vi "Wave1D_Solver.vi"(0 "F(t, x)":dbl[][](array[numeric]), 1 "Initial Value":dbl[](array[numeric]), 2 "Initial Derivative":dbl[](array[numeric]), 5 "k":dbl=1.0, 7 "a":dbl, 9 "Domain":T2={"t"={"initial t"=0.0, "final t"=1.0, "# of t-points"=11}, "x"={"start x"=0.0, "end x"=1.0, "# of x-points"=11}}, 11 "error in (no error)":errorcluster, 12 "Boundary Condition":cluster{"type":T1, "Value":dbl[]}[](array[cluster]) {"type" items=["Dirichlet", "Neumann"]}) -> (4 "U(t, x)":dbl[][](array[numeric]), 15 "error out":errorcluster)   [LabVIEW 2017, in "NI_PDE.lvlib"]
uses:
  <vilib>/gmath/NI_PDE.lvlib
  <vilib>/gmath/pde.llb/Common/PDE_BC Type.ctl
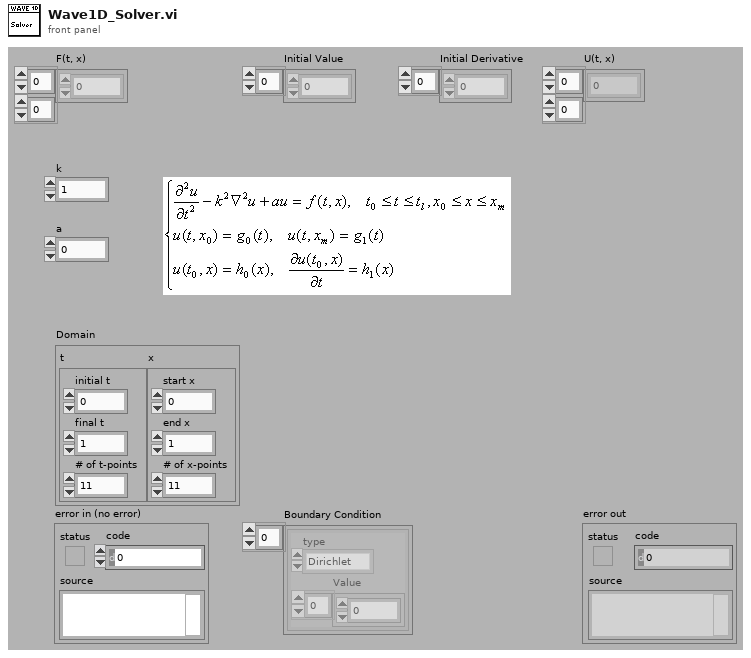
[diagram p1: front panel]
types:
  T1 = typedef "NI_PDE.lvlib/PDE_BC Type.ctl" = i32
  T2 = cluster{"t":cluster{"initial t":dbl, "final t":dbl, "# of t-points":i32}, "x":cluster{"start x":dbl, "end x":dbl, "# of x-points":i32}}
  T3 = typedef "NI_PDE.lvlib/Wave1D_Data.ctl" = cluster{"PDE":cluster{"k":dbl, "a":dbl, "F(t, x)":dbl[][]}, "Domain":cluster{"t":cluster{"initial t":dbl, "final t":dbl, "# of t-points":i32}, "x":cluster{"start x":dbl, "end x":dbl, "# of x-points":i32}, "delta":cluster{"delta t":dbl, "delta x":dbl}}, "BC":cluster{"Start X":cluster{"type":T1, "Value":dbl[]}, "End X":cluster{"type":T1, "Value":dbl[]}}, "IC":cluster{"Value":dbl[], "Derivative":dbl[]}, "A":cluster{"Sub Diag":dbl[], "Diag":dbl[], "Super Diag":dbl[], "A":T4}, "LU of A":cluster{"L":dbl[], "U":cluster{"Diag":dbl[], "Super Diag":dbl[], "2nd Super Diag":dbl[]}, "Pivot":i32[]}, "State":cluster{"U":dbl[], "AU":dbl[], "Old AU":dbl[], "start index":i32, "length":i32}}
  T4 = typedef "NI_Matrix.lvlib/RealMatrix.ctl" = dbl[][]
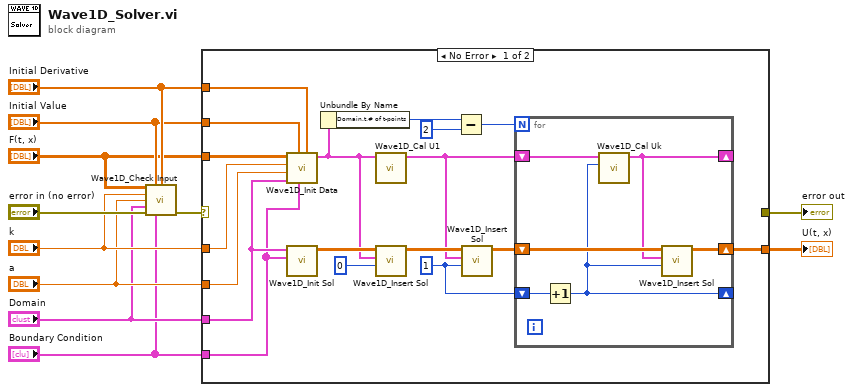
[diagram p0: block diagram]
diagram:
  n1 = call <vilib>:"Wave1D_Check Input.vi"("F(t, x)"="F(t, x)", "Initial Value"="Initial Value", "Initial Derivative"="Initial Derivative", "k"="k", "a"="a", "Domain"="Domain", "error in (no error)"="error in (no error)", "Boundary Condition"="Boundary Condition") -> ("error out"=w10:errorcluster)  [unwired: 7 out]
  n2 = case shown="No Error" w10 {
    selector: w10 -> [_ w36]
    tunnel: "Initial Derivative" -> [w28 _]
    tunnel: "Initial Value" -> [w29 _]
    tunnel: "F(t, x)" -> [w27 _]
    tunnel: "k" -> [w26 _]
    tunnel: "a" -> [w25 _]
    tunnel: "Domain" -> [w24 _]
    tunnel: "Boundary Condition" -> [w23 _]
    tunnel: [w18 _] -> w2
    tunnel: [_ w36] -> w1
    frame No Error {
      w12 = 1 ("time step")
      n3 = call <vilib>:"Wave1D_Init Data.vi"("Initial Derivative"=w28, "Boundary Condition"=w23, "Initial Value"=w29, "Domain"=w24, "a"=w25, "k"=w26, "F(t, x)"=w27) -> ("Wave1D Data"=w13:T3)  [unwired: 4 out]
      n4 = call <vilib>:"Wave1D_Init Sol.vi"("Boundary Condition"=w23, "Domain"=w24) -> ("U(t, x)"=w22:dbl[][])  [unwired: 9 out]
      n5 = Unbundle By Name(w13) -> ("Domain.t.# of t-points"=w16:i32)
      n6 = call <vilib>:"Wave1D_Cal U1.vi"("Wave1D Data In"=w13) -> ("Wave1D Data Out"=w17:T3)  [unwired: 10 out]
      n7 = call <vilib>:"Wave1D_Insert Sol.vi"("time step"=0, "Wave1D Data"=w13, "U(t, x) In"=w22) -> ("U(t, x) Out"=w20:dbl[][])  [unwired: 8 out]
      n8 = Subtract(x=w16, y=2) -> (x-y=w15:i32)
      n9 = call <vilib>:"Wave1D_Insert Sol.vi"("time step"=w12, "Wave1D Data"=w17, "U(t, x) In"=w20) -> ("U(t, x) Out"=w19:dbl[][])  [unwired: 8 out]
      n10 = for {
        N: w15 -> [_]
        shift-right: [w34] -> w18
        shift-left: w19 -> [w35]
        shift-right: [w32] -> _
        shift-left: w17 -> [w33]
        shift-right: [w30] -> _
        shift-left: w12 -> [w31]
        n11 = Increment(x=w31) -> (x+1=w30:i32)
        n12 = call <vilib>:"Wave1D_Cal Uk.vi"("time step"=w30, "Wave1D Data In"=w33) -> ("Wave1D Data Out"=w32:T3)  [unwired: 9 out]
        n13 = call <vilib>:"Wave1D_Insert Sol.vi"("time step"=w30, "Wave1D Data"=w32, "U(t, x) In"=w35) -> ("U(t, x) Out"=w34:dbl[][])  [unwired: 8 out]
      }
    }
    frame Error {
    }
  }
  "U(t, x)" <- w2
  "error out" <- w1
